vi "ni579x Load Characterization Data (Single Channel).vi"(0 "Register Bus":refnum<class "ni579x Register Bus v1 Host.lvclass">=refnum, 1 "scope":string(combo)="rx", 5 "start address":u32 format="%x", 7 "EEPROM Data Section":T4, 11 "Error In":errorcluster) -> (3 "EEPROM Header":T7 {"Product Code" format="%x"; "Checksum" format="%x"}, 4 "Register Bus (out)":refnum<class "ni579x Register Bus v1 Host.lvclass">, 6 "EEPROM Calibration Header":T6={"Checksum"=0, "Date"=timestamp(0 s since 1904-01-01), "Temperature"=0.0, "Misc. Info"="", "Pointer to Device Data Header"=0, "Number of Reserved Bytes"=28} {"Checksum" format="%x"}, 8 "Device Data Header":T5={"Checksum"=0, "Number of Channels"=0, "Number of Attenuations"=[], "Number of Attenuator Settings"=[], "Number of Gain Settings"=[], "Pointer to Cal Data"=[], "Number of Reserved Bytes"=7, "Number of Frequencies"=[]} {"Checksum" format="%x"}, 10 "Characterization Data":T1 {"Frequencies [Hz]" format="%#_6p"}, 15 "Error Out":errorcluster)   [LabVIEW 2015]
doc: "Reads characterization data from the on-device EEPROM and returns headers and characterization data for the specified channel.\n\n<B>Input Parameters</B>\n\n<B>Register Bus</B> The Register Bus object created by the ni579x Open VI and used as the session handle for the NI-579x Configuration Design Library.\n\n<B>scope</B> The channel to read characterization data for. The options are \"rx\" and \"tx\".\n\n<B>start address</B> The start offset of the data in the EEPROM.\n\n<B>EEPROM Data Section</B> The EEPROM can contain characterization data measured and calculated by the manufacturer (the Factory Data) as well as data measured and calculated by the user (the User Data).\n\n<B>Output Parameters</B>\n\n<B>Register Bus (out)</B> The Register Bus object created by the ni579x Open VI and used as the session handle for the NI-579x Configuration Design Library.\n\n<B>EEPROM Header</B> Header information for the entire EEPROM.\n\n<B>EEPROM Calibration Header</B> Header information describing the calibration sections.\n\n<B>Device Data Header</B> Header information describing the device characterization data sections.\n\n<B>Characterization Data</B> Characterization data for the specified channel."
uses:
  <instrlib>/ni579x/Register Bus/v1/Host/ni579x Register Bus v1 Host.lvclass
  <instrlib>/ni579x/Config/v1/Shared/Types/EEPROM/ni579x EEPROM Header.ctl
  <instrlib>/ni579x/Config/v1/Shared/Types/EEPROM/ni579x EEPROM Calibration Header.ctl
  <instrlib>/ni579x/Config/v1/Shared/Types/EEPROM/ni579x EEPROM Device Data Header.ctl
  <instrlib>/ni579x/Config/v1/Shared/Types/EEPROM/ni579x EEPROM Data Section.ctl
  <instrlib>/ni579x/Config/v1/Shared/Types/ni579x Characterization Data.ctl
  <instrlib>/ni579x/Config/v1/Shared/Types/ni579x IQ Imbalance.ctl
  <instrlib>/ni579x/Config/v1/Shared/Types/ni579x Gain to Attenuation Mapping.ctl
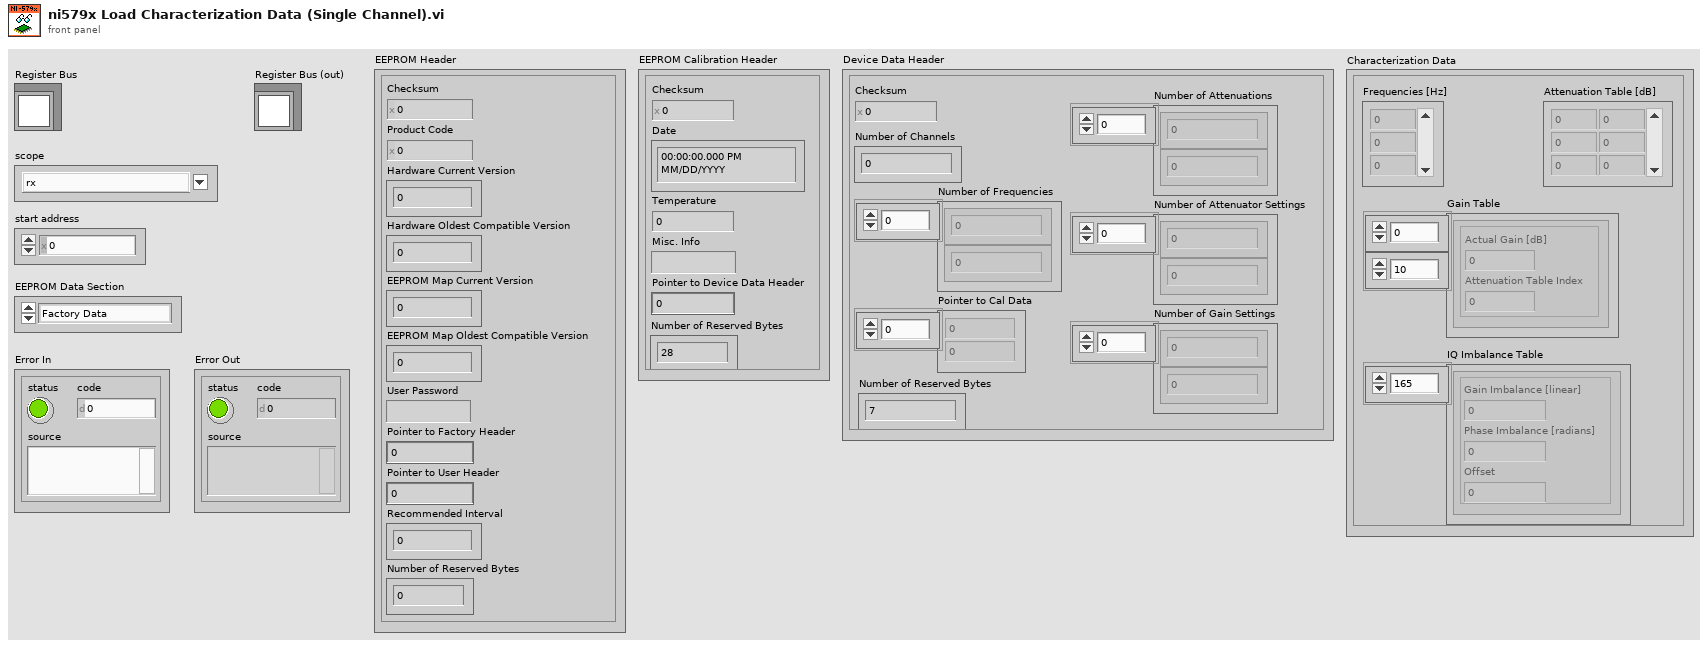
[diagram p1: front panel]
types:
  T1 = typedef "ni579x Characterization Data.ctl" = cluster{"Attenuation Table [dB]":dbl[][], "Frequencies [Hz]":dbl[], "IQ Imbalance Table":T2[], "Gain Table":T3[][]}
  T2 = typedef "ni579x IQ Imbalance.ctl" = cluster{"Gain Imbalance [linear]":dbl, "Phase Imbalance [radians]":dbl, "Offset":cdb}
  T3 = typedef "ni579x Gain to Attenuation Mapping.ctl" = cluster{"Actual Gain [dB]":dbl, "Attenuation Table Index":i32}
  T4 = typedef "ni579x EEPROM Data Section.ctl" = enum16{"Factory Data", "User Data"}
  T5 = typedef "ni579x EEPROM Device Data Header.ctl" = cluster{"Checksum":u32, "Number of Channels":u8, "Number of Attenuations":u16[], "Number of Attenuator Settings":u8[], "Number of Gain Settings":u8[], "Pointer to Cal Data":u32[], "Number of Reserved Bytes":i32, "Number of Frequencies":u16[]}
  T6 = typedef "ni579x EEPROM Calibration Header.ctl" = cluster{"Checksum":u32, "Date":timestamp, "Temperature":sgl, "Misc. Info":string, "Pointer to Device Data Header":u32, "Number of Reserved Bytes":i32}
  T7 = typedef "ni579x EEPROM Header.ctl" = cluster{"Checksum":u32, "Product Code":u16, "Hardware Current Version":u16, "Hardware Oldest Compatible Version":u16, "EEPROM Map Current Version":u16, "EEPROM Map Oldest Compatible Version":u16, "User Password":string, "Pointer to Factory Header":u32, "Pointer to User Header":u32, "Recommended Interval":u16, "Number of Reserved Bytes":i32}
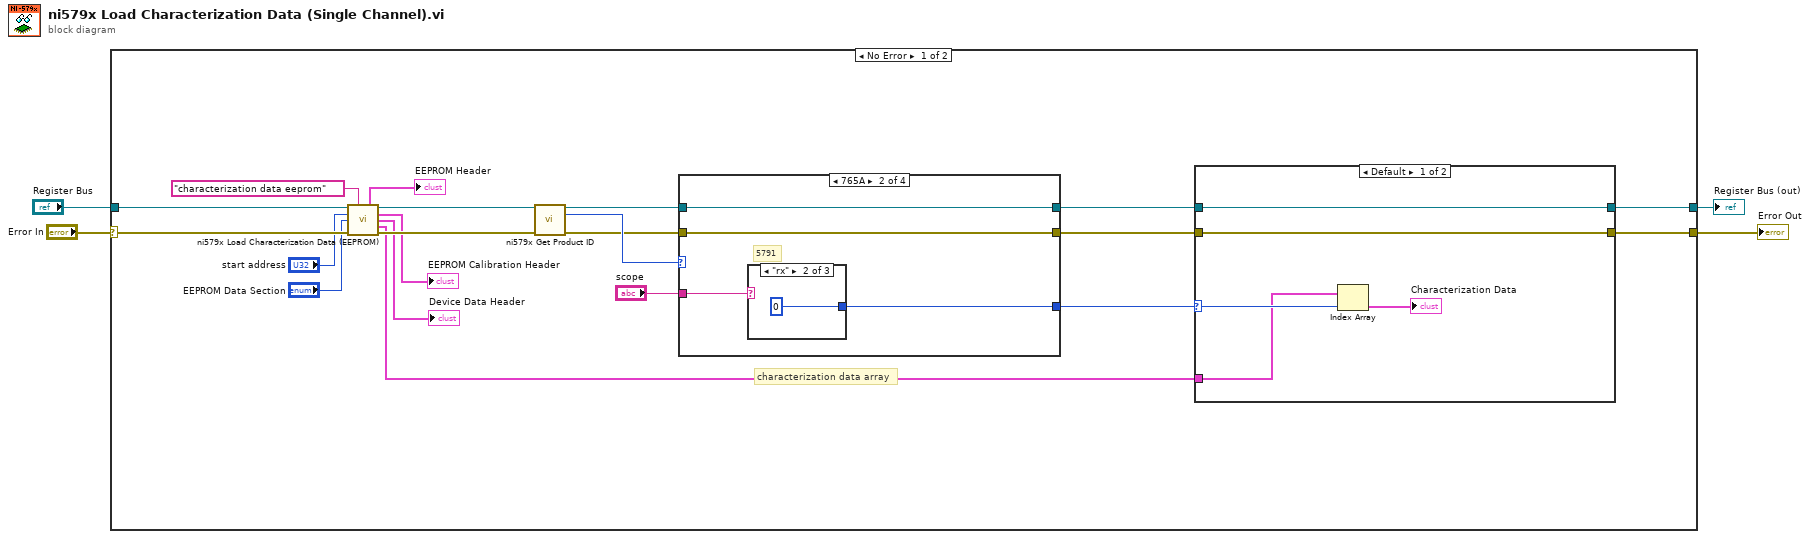
[diagram p0: block diagram]
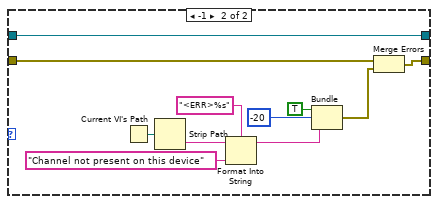
[diagram p2: hidden frame]
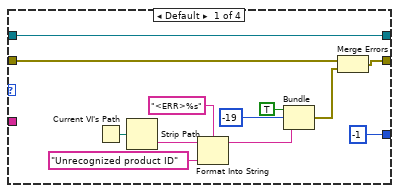
[diagram p3: hidden frame]
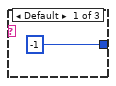
[diagram p4: hidden frame]
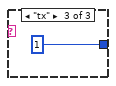
[diagram p5: hidden frame]
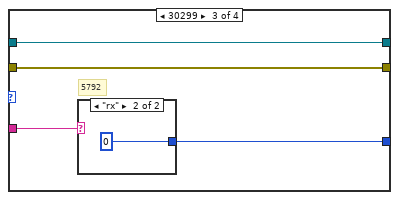
[diagram p6: hidden frame]
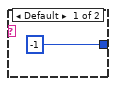
[diagram p7: hidden frame]
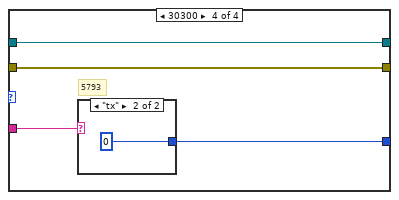
[diagram p8: hidden frame]
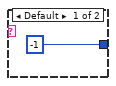
[diagram p9: hidden frame]
diagram:
  n1 = case shown="No Error" "Error In" {
    selector: "Error In" -> [w23 w73]
    tunnel: [w6 w73] -> w3
    tunnel: "Register Bus" -> [w24 w72]
    tunnel: [w5 w72] -> w1
    frame No Error {
      # "characterization data array"
      n2 = call <instrlib>:"ni579x Load Characterization Data (EEPROM).vi"("Register Bus"=w24, "scope"="characterization data eeprom", "start address"="start address", "EEPROM Data Section"="EEPROM Data Section", "Error In"=w23) -> ("EEPROM Header"=→"EEPROM Header":T7, "Register Bus (out)"=w18:refnum<class "ni579x Register Bus v1 Host.lvclass">, "EEPROM Calibration Header"=→"EEPROM Calibration Header":T6, "Device Data Header"=→"Device Data Header":T5, "Characterization Data"=w8:T1[], "Error Out"=w17:errorcluster)  [unwired: 5 in]
      n3 = call <instrlib>:"ni579x Get Product ID.vi"("Register Bus"=w18, "Error In"=w17) -> ("Register Bus (out)"=w11:refnum<class "ni579x Register Bus v1 Host.lvclass">, "product ID"=w14:u16, "Error Out"=w12:errorcluster)  [unwired: 11 in]
      n4 = case shown="765A" w14 {
        tunnel: "scope" -> [_ w56 w63 w69]
        tunnel: [-1 w55 w62 w68] -> w10
        tunnel: w12 -> [w44 w54 w60 w66]
        tunnel: w11 -> [w43 w53 w61 w67]
        tunnel: [w42 w54 w60 w66] -> w9
        tunnel: [w43 w53 w61 w67] -> w7
        frame Default {
          n5 = Current VI's Path() -> (path=w46:path)
          n6 = Strip Path(path=w46) -> (name=w47:string)  [unwired: 1 out]
          n7 = Format Into String(format string="<ERR>%s", initial string=w47, "Unrecognized product ID" ("input 1")) -> (resulting string=w48:string)  [unwired: 1 in, 1 out]
          n8 = Bundle("status"=TRUE, "code"=-19, w48) -> (w49:cluster{"status":bool, "code":i32, string})  [unwired: 1 in]
          n9 = Merge Errors(w44, w49) -> (w42:errorcluster)
        }
        frame 30298 {
          # "5791"
          n10 = case shown="\"rx\"" w56 {
            tunnel: [-1 0 1] -> w55
            frame Default {
            }
            frame "rx" {
            }
            frame "tx" {
            }
          }
        }
        frame 30299 {
          # "5792"
          n11 = case shown="\"rx\"" w63 {
            tunnel: [-1 0] -> w62
            frame Default {
            }
            frame "rx" {
            }
          }
        }
        frame 30300 {
          # "5793"
          n12 = case shown="\"tx\"" w69 {
            tunnel: [-1 0] -> w68
            frame Default {
            }
            frame "tx" {
            }
          }
        }
      }
      n13 = case shown="Default" w10 {
        selector: w10 -> [w29 _]
        tunnel: w9 -> [w26 w32]
        tunnel: w8 -> [w28 _]
        tunnel: [w26 w31] -> w6
        tunnel: w7 -> [w25 w30]
        tunnel: [w25 w30] -> w5
        frame Default {
          n14 = Index Array(array=w28, index=w29) -> (element=→"Characterization Data":T1)
        }
        frame -1 {
          n15 = Current VI's Path() -> (path=w39:path)
          n16 = Strip Path(path=w39) -> (name=w38:string)  [unwired: 1 out]
          n17 = Format Into String(format string="<ERR>%s", initial string=w38, "Channel not present on this device" ("input 1")) -> (resulting string=w37:string)  [unwired: 1 in, 1 out]
          n18 = Bundle("status"=TRUE, "code"=-20, w37) -> (w36:cluster{"status":bool, "code":i32, string})  [unwired: 1 in]
          n19 = Merge Errors(w32, w36) -> (w31:errorcluster)
        }
      }
    }
    frame Error {
    }
  }
  "Register Bus (out)" <- w1
  "Error Out" <- w3
